vi "Create_pop_arrays.vi"(8 "Zero ensemble in":dbl[](array[numeric]), 9 "Zero ensemble area in":dbl, 10 "Normalized I in":dbl[](array[numeric]), 11 "Saturation Polarization":dbl) -> (0 "Zero ensemble out":dbl[](array[numeric]), 1 "rho- array out":dbl[](array[numeric]), 2 "rho0 array out":dbl[](array[numeric]), 3 "rho+ array out":dbl[](array[numeric]))   [LabVIEW 2018]
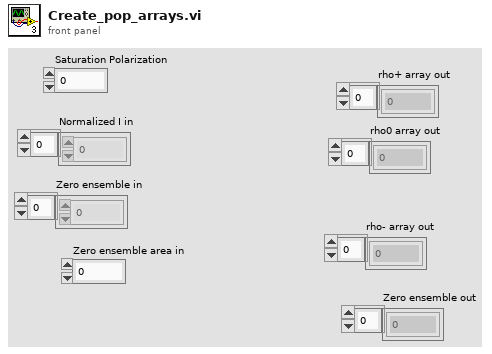
[diagram p1: front panel]
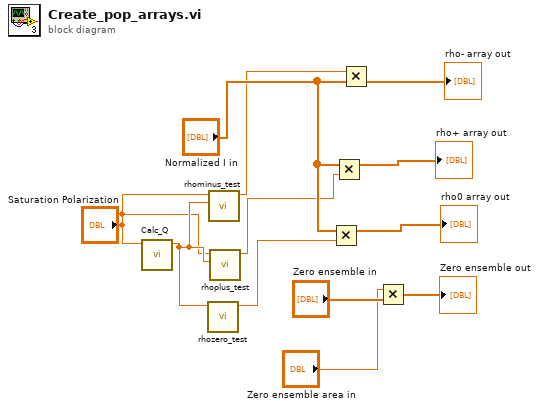
[diagram p0: block diagram]
diagram:
  n1 = call "Calc_Q.vi"("P"="Saturation Polarization") -> ("Q"=w8:dbl)  [unwired: 10 in]
  n2 = call "rhozero_test.vi"("Q in"=w8) -> ("rho0 value out"=w3:dbl)  [unwired: 10 in]
  n3 = call "rhominus_test.vi"("Q in"=w8, "P in"="Saturation Polarization") -> ("rho+ value out"=w6:dbl)  [unwired: 9 in]
  n4 = call "rhoplus_test.vi"("Q in"=w8, "P in"="Saturation Polarization") -> ("rho+ value out"=w5:dbl)  [unwired: 9 in]
  n5 = Multiply(x="Normalized I in", y=w3) -> (x*y=→"rho0 array out":dbl[])
  n6 = Multiply(x="Normalized I in", y=w5) -> (x*y=→"rho+ array out":dbl[])
  n7 = Multiply(x=w6, y="Normalized I in") -> (x*y=→"rho- array out":dbl[])
  n8 = Multiply(x="Zero ensemble area in", y="Zero ensemble in") -> (x*y=→"Zero ensemble out":dbl[])
